vi "Configure Measurement Cursors.vi"(11 "State in":T1={"Graph Visible Items"={"Plot Legend"=FALSE, "Scale Legend"=FALSE, "Graph Palette"=FALSE, "Cursor Legend"=FALSE, "X Scrollbar"=FALSE}, "View Table"=FALSE, "Table Visible Items"={"Vertical Scrollbar"=FALSE, "Horizontal Scrollbar"=FALSE, "Row Headers"=FALSE, "Column Headers"=FALSE, "Vertical Lines"=FALSE, "Horizontal Lines"=FALSE}, "Header Font"={"Font Name"="", "Size"=0, "Bold"=FALSE, "Italic"=FALSE, "Underline"=FALSE, "Strikeout"=FALSE, "Color"=0}, "Cell Font"={"Font Name"="", "Size"=0, "Bold"=FALSE, "Italic"=FALSE, "Underline"=FALSE, "Strikeout"=FALSE, "Color"=0}, "Description and Tip..."={"Description"="", "Tip"=""}, "Moveable Splitter Position"=0, "Measurement Cursor Configuration"={"relative to t0"={"enable relative time"=FALSE, "Relative times (DT)"=[], "color"=0}, "range"={"enable range"=FALSE, "T1"=0.0, "T2"=0.0, "Fixed interval (T2-T1)"=0.0, "T1 color"=0, "T2 color"=0, "enable shading"=FALSE}, "periodic"={"enable periodic"=FALSE, "First event (E1)"=0.0, "Number events (Ei)"=0, "Event spacing (s)"=0.0, "First color"=0, "Events color"=0}, "absolute timestamp"={"enable absolute"=FALSE, "Timestamps (TS)"=[], "color"=0}}, "X Increment"=0.0, "X Scale"={"Label Visible"=FALSE, "Label Text"="", "Time Mode"=enum."Relative", "Format String"=""}, "Y Scale"={"Label Visible"=FALSE, "Label Text"="", "Scaling"=enum."Engineering Units", "Format String"=""}, "Colors"={"background"=16777215, "major grid"=8355711, "minor grid"=12632256, "font"=0}, "Cursors"={"List"=[], "Tags"=[]}, "Plots"=[], "Plot Color Wheel"=[3381759, 32768, 982784, 4375295, 13827953, 13457919, 16757522, 4343295, 16728758, 12095254], "registered user events"=variant} caption="State") -> (1 "OK":bool=TRUE, 3 "State out":T1={"Graph Visible Items"={"Plot Legend"=FALSE, "Scale Legend"=FALSE, "Graph Palette"=FALSE, "Cursor Legend"=FALSE, "X Scrollbar"=FALSE}, "View Table"=FALSE, "Table Visible Items"={"Vertical Scrollbar"=FALSE, "Horizontal Scrollbar"=FALSE, "Row Headers"=FALSE, "Column Headers"=FALSE, "Vertical Lines"=FALSE, "Horizontal Lines"=FALSE}, "Header Font"={"Font Name"="", "Size"=0, "Bold"=FALSE, "Italic"=FALSE, "Underline"=FALSE, "Strikeout"=FALSE, "Color"=0}, "Cell Font"={"Font Name"="", "Size"=0, "Bold"=FALSE, "Italic"=FALSE, "Underline"=FALSE, "Strikeout"=FALSE, "Color"=0}, "Description and Tip..."={"Description"="", "Tip"=""}, "Moveable Splitter Position"=0, "Measurement Cursor Configuration"={"relative to t0"={"enable relative time"=TRUE, "Relative times (DT)"=[10.0], "color"=0}, "range"={"enable range"=TRUE, "T1"=0.0, "T2"=0.0, "Fixed interval (T2-T1)"=0.0, "T1 color"=0, "T2 color"=0, "enable shading"=FALSE}, "periodic"={"enable periodic"=TRUE, "First event (E1)"=0.0, "Number events (Ei)"=0, "Event spacing (s)"=0.0, "First color"=0, "Events color"=0}, "absolute timestamp"={"enable absolute"=TRUE, "Timestamps (TS)"=[timestamp(3458182847.281708 s since 1904-01-01), timestamp(3458182851.510322 s since 1904-01-01)], "color"=0}}, "X Increment"=0.0, "X Scale"={"Label Visible"=FALSE, "Label Text"="", "Time Mode"=enum."Relative", "Format String"=""}, "Y Scale"={"Label Visible"=FALSE, "Label Text"="", "Scaling"=enum."Engineering Units", "Format String"=""}, "Colors"={"background"=16777215, "major grid"=8355711, "minor grid"=12632256, "font"=0}, "Cursors"={"List"=[], "Tags"=[]}, "Plots"=[], "Plot Color Wheel"=[3381759, 32768, 982784, 4375295, 13827953, 13457919, 16757522, 4343295, 16728758, 12095254], "registered user events"=variant} caption="State")   [LabVIEW 2017, in "Waveforms with Cursors.xctl"]
doc: "Dialog for cursor configuration."
uses:
  <vilib>/addons/_XControls/Waveforms with Cursors/Waveforms with Cursors.xctl
  <vilib>/addons/_XControls/Waveforms with Cursors/Controls/State.ctl
  <vilib>/Utility/miscctls.llb/LVFontTypeDef.ctl
  <vilib>/addons/_XControls/Waveforms with Cursors/Controls/Waveform Cursor Configuration.ctl
panel:
  in  "enable shading":bool=TRUE
  in  "X2 color":u32(colorbox)
  in  "X1 color":u32(colorbox)
  in  "Fixed interval":dbl=-1.0 format="%#_4p"
  in  "enable range":bool=TRUE
  in  "Stop (t2)":dbl=0.075 format="%#_4p"
  in  "Start (t1)":dbl=0.025 format="%#_4p"
  in  "enable XY":bool=TRUE
  in  "Position (t)":dbl[](array[numeric])=[0.01] min=0.0 step=1.0 format="%#_6p"
  in  "XY color":u32(colorbox)
  in  "1X color":u32(colorbox)
  in  "enable timestamp":bool=TRUE
  in  "Timestamp (ts)":timestamp[](array[timestamp])=[timestamp(3458199600 s since 1904-01-01)]
  in  "Center color":u32(colorbox)
  in  "Sideband color":u32(colorbox)
  in  "Events":i32=2 min=1 max=9 step=1
  in  "enable periodic":bool=TRUE
  in  "Fixed interval":dbl=0.05 step=1.0 format="%#_4p"
  in  "Event (e1)":dbl=0.025 min=0.001 step=0.001 format="%#_4p"
  in  "Cancel":bool
  in  "OK":bool
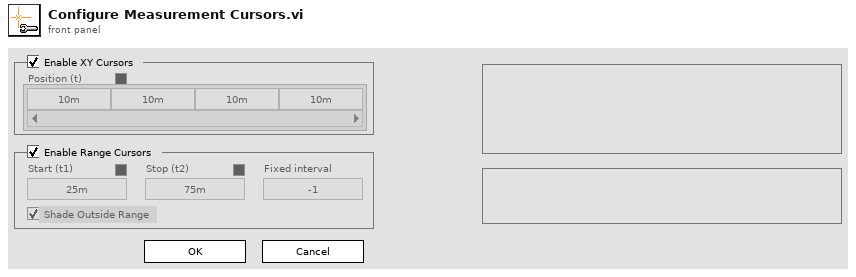
[diagram p1: front panel]
types:
  T1 = typedef "Waveforms with Cursors.xctl/State.ctl" = cluster{"Graph Visible Items":cluster{"Plot Legend":bool, "Scale Legend":bool, "Graph Palette":bool, "Cursor Legend":bool, "X Scrollbar":bool}, "View Table":bool, "Table Visible Items":cluster{"Vertical Scrollbar":bool, "Horizontal Scrollbar":bool, "Row Headers":bool, "Column Headers":bool, "Vertical Lines":bool, "Horizontal Lines":bool}, "Header Font":T2, "Cell Font":T2, "Description and Tip...":cluster{"Description":string, "Tip":string}, "Moveable Splitter Position":i32, "Measurement Cursor Configuration":T3, "X Increment":dbl, "X Scale":cluster{"Label Visible":bool, "Label Text":string, "Time Mode":enum16{"Relative", "Absolute"}, "Format String":string}, "Y Scale":cluster{"Label Visible":bool, "Label Text":string, "Scaling":enum16{"Engineering Units", "Voltage"}, "Format String":string}, "Colors":cluster{"background":u32, "major grid":u32, "minor grid":u32, "font":u32}, "Cursors":cluster{"List":cluster{"Name":string, "Color":u32, "Style":i32, "Point Style":u8, "Name Visible":bool, "Allow Drag":bool, "Cursor Mode":u32, "Plot":i32, "Index":i32, "Position":cluster{"X":dbl, "Y":dbl}, "X Scale":u32, "Y Scale":u32, "Watch Plots":i32[], "Watch All Plots":bool, "Plot Area":i32, "Label Offset":cluster{"X":dbl, "Y":dbl}}[], "Tags":variant[]}, "Plots":cluster{"Name":string, "Line Color":u32, "Line Style":u8, "Line Width":u8, "Fill/Point Color":u32, "Point Style":u8, "Fill To":i16, "Interpolation":u8, "Anti-aliased":bool}[], "Plot Color Wheel":u32[], "registered user events":variant}
  T2 = typedef "LVFontTypeDef.ctl" = cluster{"Font Name":string, "Size":u16, "Bold":bool, "Italic":bool, "Underline":bool, "Strikeout":bool, "Color":u32}
  T3 = typedef "Waveforms with Cursors.xctl/Waveform Cursor Configuration.ctl" = cluster{"relative to t0":cluster{"enable relative time":bool, "Relative times (DT)":dbl[], "color":u32}, "range":cluster{"enable range":bool, "T1":dbl, "T2":dbl, "Fixed interval (T2-T1)":dbl, "T1 color":u32, "T2 color":u32, "enable shading":bool}, "periodic":cluster{"enable periodic":bool, "First event (E1)":dbl, "Number events (Ei)":i32, "Event spacing (s)":dbl, "First color":u32, "Events color":u32}, "absolute timestamp":cluster{"enable absolute":bool, "Timestamps (TS)":timestamp[], "color":u32}}
  T4 = cluster{"enable relative time":bool, "Relative times (DT)":dbl[], "color":u32}
  T5 = cluster{"enable absolute":bool, "Timestamps (TS)":timestamp[], "color":u32}
  T6 = cluster{"enable periodic":bool, "First event (E1)":dbl, "Number events (Ei)":i32, "Event spacing (s)":dbl, "First color":u32, "Events color":u32}
  T7 = cluster{"enable range":bool, "T1":dbl, "T2":dbl, "Fixed interval (T2-T1)":dbl, "T1 color":u32, "T2 color":u32, "enable shading":bool}
  T8 = enum8{"Enabled", "Disabled", "Disabled and Grayed Out"}
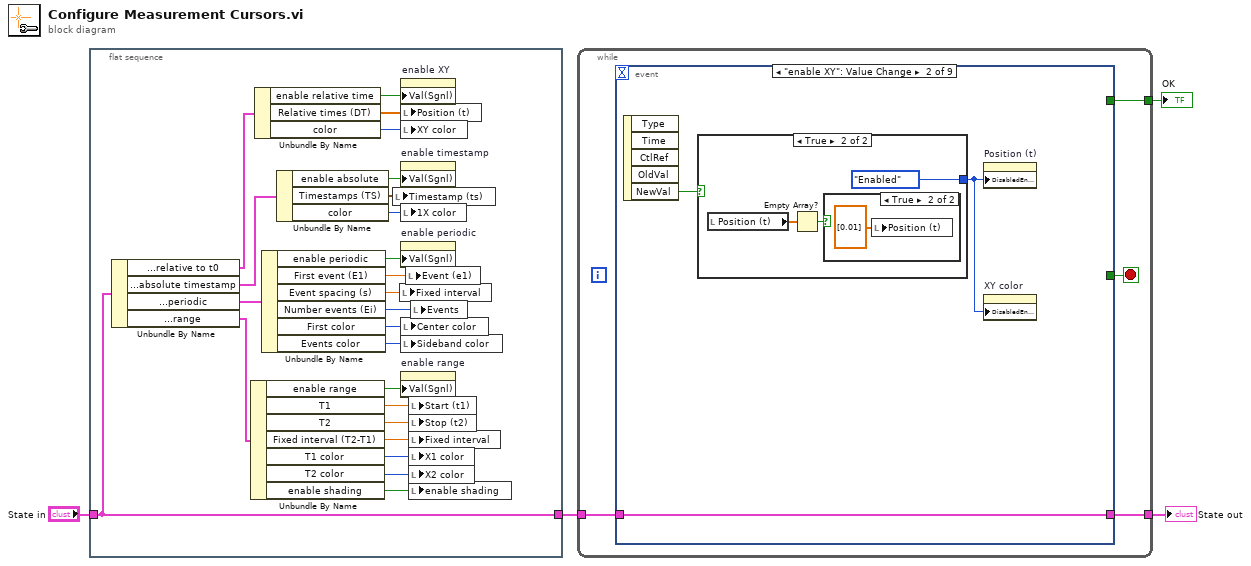
[diagram p0: block diagram]
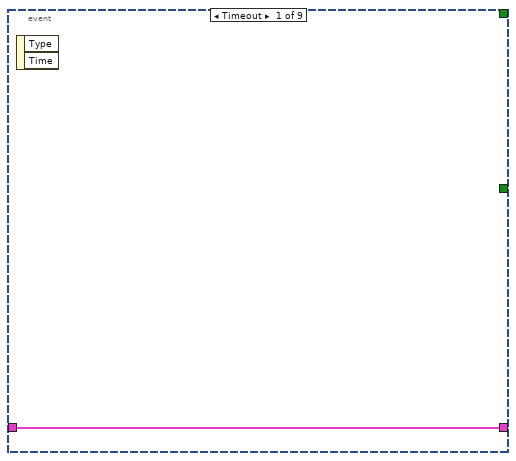
[diagram p2: hidden frame]
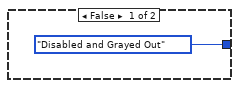
[diagram p3: hidden frame]
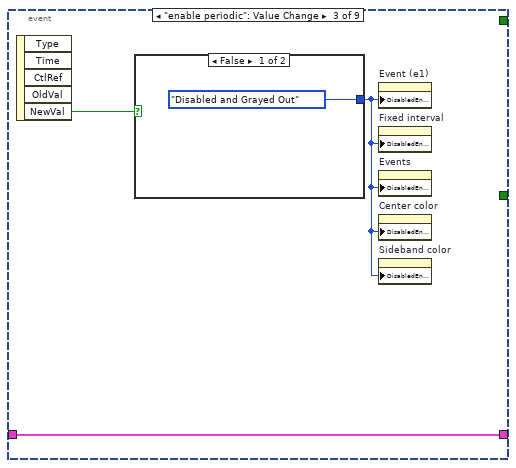
[diagram p5: hidden frame]
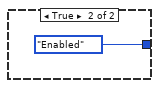
[diagram p6: hidden frame]
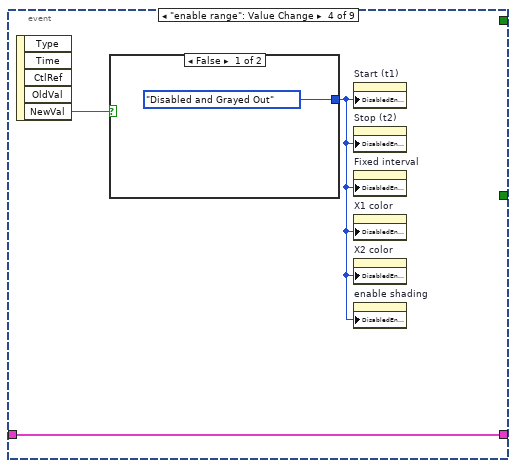
[diagram p7: hidden frame]
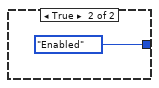
[diagram p8: hidden frame]
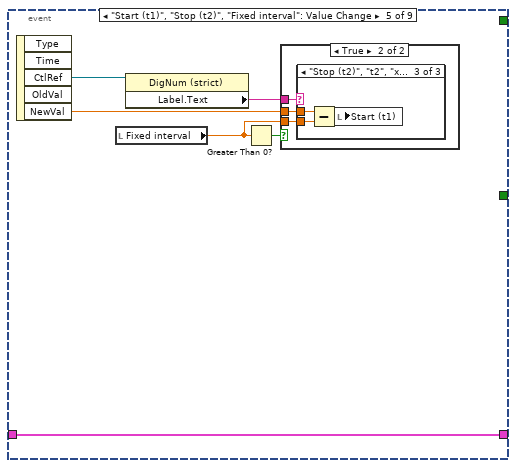
[diagram p9: hidden frame]
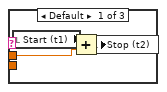
[diagram p11: hidden frame]
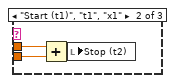
[diagram p12: hidden frame]
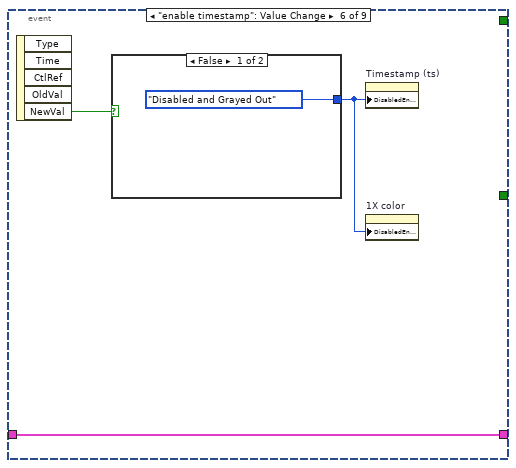
[diagram p13: hidden frame]
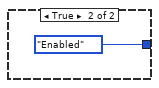
[diagram p14: hidden frame]
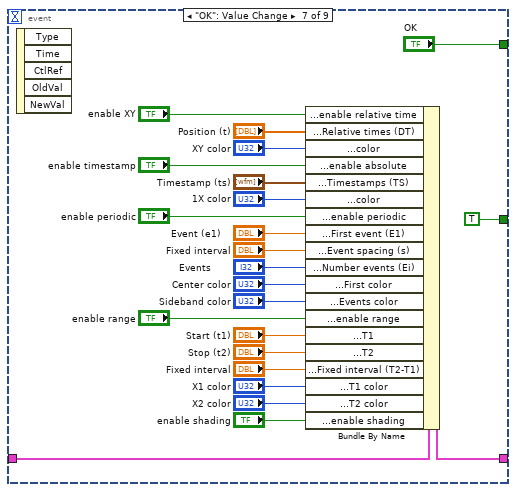
[diagram p15: hidden frame]
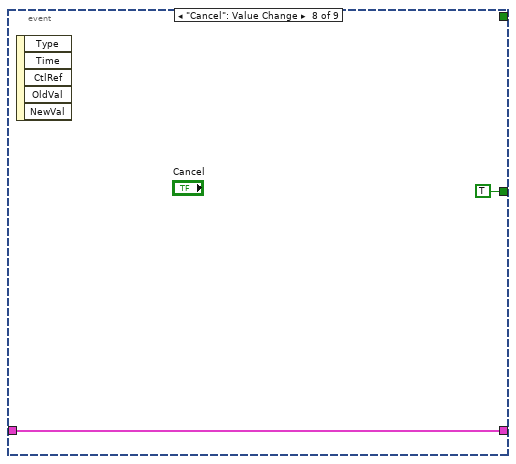
[diagram p16: hidden frame]
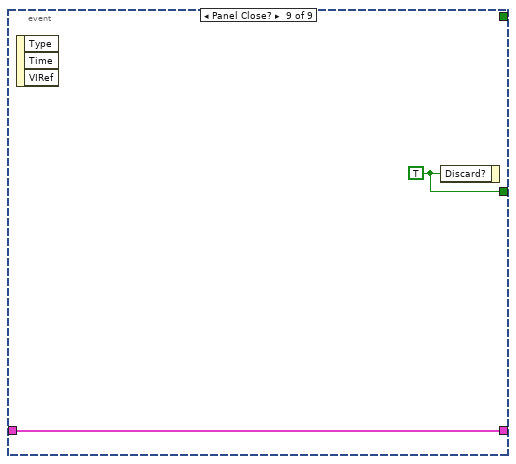
[diagram p17: hidden frame]
diagram:
  n1 = flat-sequence {
    tunnel: "State in" -> [w16]
    tunnel: [w16] -> w2
    frame #0 {
      n2 = Unbundle By Name(w16) -> ("Measurement Cursor Configuration.relative to t0"=w28:T4, "Measurement Cursor Configuration.absolute timestamp"=w26:T5, "Measurement Cursor Configuration.periodic"=w24:T6, "Measurement Cursor Configuration.range"=w20:T7)
      n3 = Unbundle By Name(w20) -> ("enable range"=w12:bool, "T1"=w19:dbl, "T2"=w18:dbl, "Fixed interval (T2-T1)"=w17:dbl, "T1 color"=w8:u32, "T2 color"=w7:u32, "enable shading"=w5:bool)
      n4 = Unbundle By Name(w28) -> ("enable relative time"=w15:bool, "Relative times (DT)"=w27:dbl[], "color"=w6:u32)
      n5 = Unbundle By Name(w24) -> ("enable periodic"=w13:bool, "First event (E1)"=w23:dbl, "Event spacing (s)"=w22:dbl, "Number events (Ei)"=w21:i32, "First color"=w10:u32, "Events color"=w9:u32)
      n6 = Unbundle By Name(w26) -> ("enable absolute"=w14:bool, "Timestamps (TS)"=w25:timestamp[], "color"=w11:u32)
      n7 = local write "Timestamp (ts)"(w25) -> ()
      n8 = local write "Fixed interval"(w22) -> ()
      n9 = property on="enable XY" class="Bool (strict)"("Val(Sgnl)"=w15) -> ()  [unwired: 2 in, 2 out]
      n10 = local write "Position (t)"(w27) -> ()
      n11 = local write "XY color"(w6) -> ()
      n12 = property on="enable timestamp" class="Bool (strict)"("Val(Sgnl)"=w14) -> ()  [unwired: 2 in, 2 out]
      n13 = local write "1X color"(w11) -> ()
      n14 = property on="enable periodic" class="Bool (strict)"("Val(Sgnl)"=w13) -> ()  [unwired: 2 in, 2 out]
      n15 = local write "Center color"(w10) -> ()
      n16 = local write "Sideband color"(w9) -> ()
      n17 = property on="enable range" class="Bool (strict)"("Val(Sgnl)"=w12) -> ()  [unwired: 2 in, 2 out]
      n18 = local write "Event (e1)"(w23) -> ()
      n19 = local write "Start (t1)"(w19) -> ()
      n20 = local write "Stop (t2)"(w18) -> ()
      n21 = local write "Fixed interval"(w17) -> ()
      n22 = local write "X1 color"(w8) -> ()
      n23 = local write "X2 color"(w7) -> ()
      n24 = local write "enable shading"(w5) -> ()
      n25 = local write "Events"(w21) -> ()
    }
  }
  n26 = while {
    tunnel: w2 -> [w30]
    tunnel: [w31] -> w4
    tunnel: [w29] -> w1
    stop <- w32 stop-if-true
    n27 = event shown="[1] \"enable XY\": Value Change" {
      selector: _ -> [_ _ _ _ _ _ _ _ _]
      dyn-events: _ -> [_ _ _ _ _ _ _ _ _]
      timeout: _ -> [_ _ _ _ _ _ _ _ _]
      tunnel: [_ _ _ _ _ _ TRUE TRUE w100] -> w32
      tunnel: [w33 w35 w43 w48 w57 w71 w86 w98 w101] -> w31
      tunnel: w30 -> [w33 w35 w43 w48 w57 w71 w87 w98 w101]
      tunnel: [_ _ _ _ _ _ "OK" _ _] -> w29
      event Timeout {
        n28 = event-data() -> ()  [unwired: 1 in, 2 out]
      }
      event "enable XY": Value Change {
        n29 = event-data() -> ("NewVal"=w36:bool)  [unwired: 1 in, 4 out]
        n30 = case shown="True" w36 {
          tunnel: [T8."Disabled and Grayed Out" ("Disabled") T8."Enabled" ("Disabled")] -> w34
          frame False {
          }
          frame True {
            n31 = local read "Position (t)"() -> (w39:dbl[])
            n32 = Empty Array?(array=w39) -> (empty?=w38:bool)
            n33 = case shown="True" w38 {
              frame False {
              }
              frame True {
                n34 = local write "Position (t)"(dbl[] [0.01] ("Position (t)")) -> ()
              }
            }
          }
        }
        n35 = property on="Position (t)" class="Arr (strict)"("DisabledEnum"=w34) -> ()  [unwired: 2 in, 2 out]
        n36 = property on="XY color" class="ColBox"("DisabledEnum"=w34) -> ()  [unwired: 2 in, 2 out]
      }
      event "enable periodic": Value Change {
        n37 = event-data() -> ("NewVal"=w44:bool)  [unwired: 1 in, 4 out]
        n38 = case shown="False" w44 {
          tunnel: [T8."Disabled and Grayed Out" ("Disabled") T8."Enabled" ("Disabled")] -> w42
          frame False {
          }
          frame True {
          }
        }
        n39 = property on="Event (e1)" class="DigNum (strict)"("DisabledEnum"=w42) -> ()  [unwired: 2 in, 2 out]
        n40 = property on="Fixed interval" class="DigNum (strict)"("DisabledEnum"=w42) -> ()  [unwired: 2 in, 2 out]
        n41 = property on="Events" class="DigNum (strict)"("DisabledEnum"=w42) -> ()  [unwired: 2 in, 2 out]
        n42 = property on="Center color" class="ColBox"("DisabledEnum"=w42) -> ()  [unwired: 2 in, 2 out]
        n43 = property on="Sideband color" class="ColBox"("DisabledEnum"=w42) -> ()  [unwired: 2 in, 2 out]
      }
      event "enable range": Value Change {
        n44 = event-data() -> ("NewVal"=w49:bool)  [unwired: 1 in, 4 out]
        n45 = case shown="False" w49 {
          tunnel: [T8."Disabled and Grayed Out" ("Disabled") T8."Enabled" ("Disabled")] -> w47
          frame False {
          }
          frame True {
          }
        }
        n46 = property on="Start (t1)" class="DigNum (strict)"("DisabledEnum"=w47) -> ()  [unwired: 2 in, 2 out]
        n47 = property on="Stop (t2)" class="DigNum (strict)"("DisabledEnum"=w47) -> ()  [unwired: 2 in, 2 out]
        n48 = property on="Fixed interval" class="DigNum (strict)"("DisabledEnum"=w47) -> ()  [unwired: 2 in, 2 out]
        n49 = property on="X1 color" class="ColBox"("DisabledEnum"=w47) -> ()  [unwired: 2 in, 2 out]
        n50 = property on="X2 color" class="ColBox"("DisabledEnum"=w47) -> ()  [unwired: 2 in, 2 out]
        n51 = property on="enable shading" class="Bool (strict)"("DisabledEnum"=w47) -> ()  [unwired: 2 in, 2 out]
      }
      event "Start (t1)", "Stop (t2)", "Fixed interval": Value Change {
        n52 = event-data() -> ("CtlRef"=w56:refnum<vi>, "NewVal"=w54:dbl)  [unwired: 1 in, 3 out]
        n53 = local read "Fixed interval"() -> (w52:dbl)
        n54 = property class="DigNum (strict)"(reference=w56) -> ("Label.Text"=w55:string)  [unwired: 1 in, 2 out]
        n55 = Greater Than 0?(x=w52) -> (x > 0?=w53:bool)
        n56 = case shown="True" w53 {
          tunnel: w55 -> [_ w60]
          tunnel: w54 -> [_ w59]
          tunnel: w52 -> [_ w58]
          frame False {
          }
          frame True {
            n57 = case shown="\"Stop (t2)\", \"t2\", \"x2\"" w60 {
              tunnel: w59 -> [w63 w66 w69]
              tunnel: w58 -> [_ w65 w68]
              frame Default {
                n58 = local read "Start (t1)"() -> (w62:dbl)
                n59 = Add(x=w62, y=w63) -> (x+y=w61:dbl)
                n60 = local write "Stop (t2)"(w61) -> ()
              }
              frame "Start (t1)", "t1", "x1" {
                n61 = Add(x=w66, y=w65) -> (x+y=w64:dbl)
                n62 = local write "Stop (t2)"(w64) -> ()
              }
              frame "Stop (t2)", "t2", "x2" {
                n63 = Subtract(x=w69, y=w68) -> (x-y=w67:dbl)
                n64 = local write "Start (t1)"(w67) -> ()
              }
            }
          }
        }
      }
      event "enable timestamp": Value Change {
        n65 = event-data() -> ("NewVal"=w72:bool)  [unwired: 1 in, 4 out]
        n66 = case shown="False" w72 {
          tunnel: [T8."Disabled and Grayed Out" ("Disabled") T8."Enabled" ("Disabled")] -> w70
          frame False {
          }
          frame True {
          }
        }
        n67 = property on="Timestamp (ts)" class="Arr (strict)"("DisabledEnum"=w70) -> ()  [unwired: 2 in, 2 out]
        n68 = property on="1X color" class="ColBox"("DisabledEnum"=w70) -> ()  [unwired: 2 in, 2 out]
      }
      event "OK": Value Change {
        n69 = event-data() -> ()  [unwired: 1 in, 5 out]
        n70 = Bundle By Name(cluster=w87, "Measurement Cursor Configuration.relative to t0.enable relative time"="enable XY", "Measurement Cursor Configuration.relative to t0.Relative times (DT)"="Position (t)", "Measurement Cursor Configuration.relative to t0.color"="XY color", "Measurement Cursor Configuration.absolute timestamp.enable absolute"="enable timestamp", "Measurement Cursor Configuration.absolute timestamp.Timestamps (TS)"="Timestamp (ts)", "Measurement Cursor Configuration.absolute timestamp.color"="1X color", "Measurement Cursor Configuration.periodic.enable periodic"="enable periodic", "Measurement Cursor Configuration.periodic.First event (E1)"="Event (e1)", "Measurement Cursor Configuration.periodic.Event spacing (s)"="Fixed interval", "Measurement Cursor Configuration.periodic.Number events (Ei)"="Events", "Measurement Cursor Configuration.periodic.First color"="Center color", "Measurement Cursor Configuration.periodic.Events color"="Sideband color", "Measurement Cursor Configuration.range.enable range"="enable range", "Measurement Cursor Configuration.range.T1"="Start (t1)", "Measurement Cursor Configuration.range.T2"="Stop (t2)", "Measurement Cursor Configuration.range.Fixed interval (T2-T1)"="Fixed interval", "Measurement Cursor Configuration.range.T1 color"="X1 color", "Measurement Cursor Configuration.range.T2 color"="X2 color", "Measurement Cursor Configuration.range.enable shading"="enable shading") -> (w86:T1)
      }
      event "Cancel": Value Change {
        n71 = event-data() -> ()  [unwired: 1 in, 5 out]
      }
      event Panel Close? {
        w100 = TRUE ("Discard?")
        n72 = event-data() -> ()  [unwired: 1 in, 3 out]
        n73 = event-data("Discard?"=w100) -> ()  [unwired: 1 in, 1 out]
      }
    }
  }
  "State out" <- w4
  "OK" <- w1
